vi "Set Date References.vi"(8 "error in (no error)":errorcluster, 9 "Month":refnum<vi>, 10 "YYYY":refnum<vi>, 11 "Budgetizer in":refnum<class "Budgetizer.lvclass">) -> (0 "error out":errorcluster, 3 "Budgetizer out":refnum<class "Budgetizer.lvclass">)   [LabVIEW 2018, in "Budgetizer.lvclass"]
uses:
  Budgetizer.lvclass
  Budgetizer.lvclass/Budgetizer.ctl
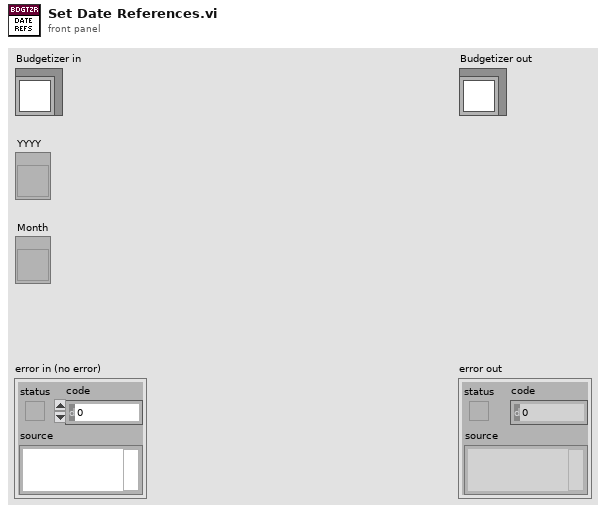
[diagram p1: front panel]
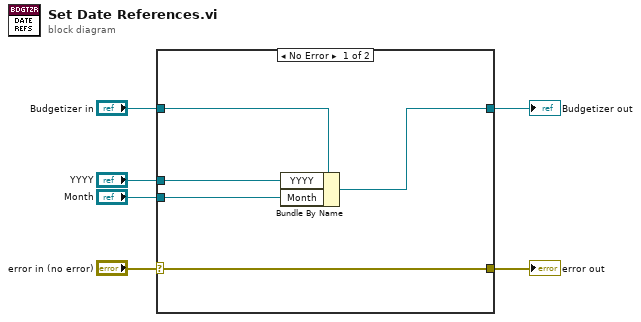
[diagram p0: block diagram]
diagram:
  n1 = case shown="No Error" "error in (no error)" {
    selector: "error in (no error)" -> [w11 w13]
    tunnel: [w11 w13] -> w5
    tunnel: [w9 w12] -> w3
    tunnel: "Budgetizer in" -> [w10 w12]
    tunnel: "Month" -> [w8 _]
    tunnel: "YYYY" -> [w7 _]
    frame No Error {
      n2 = Bundle By Name(cluster=w10, "YYYY"=w7, "Month"=w8) -> (w9:refnum<class "Budgetizer.lvclass">)
    }
    frame Error {
    }
  }
  "error out" <- w5
  "Budgetizer out" <- w3
